vi "Error Test Label Name.vi"(6 "error text in":string, 7 "reset (F)":bool, 8 "error in":errorcluster, 10 "label name":string) -> (0 "error out":errorcluster)   [LabVIEW 2020]
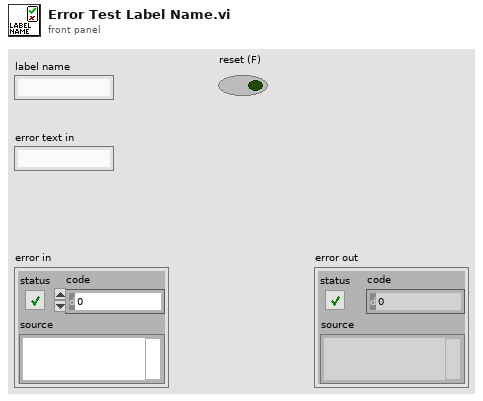
[diagram p1: front panel]
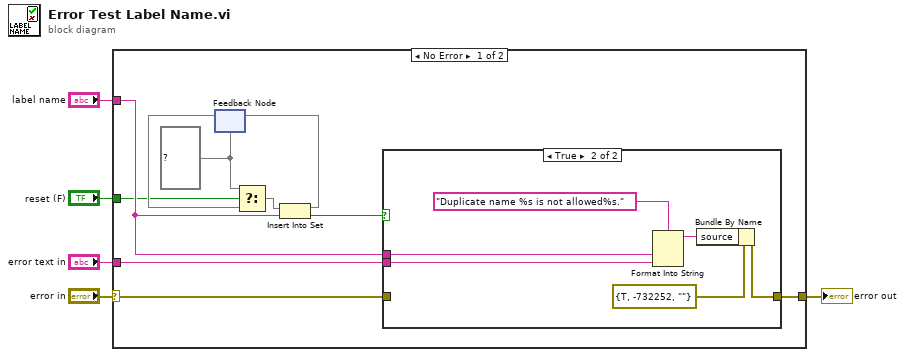
[diagram p0: block diagram]
diagram:
  n1 = case shown="No Error" "error in" {
    selector: "error in" -> [w14 w23]
    tunnel: [w13 w23] -> w4
    tunnel: "label name" -> [w15 _]
    tunnel: "reset (F)" -> [w7 _]
    tunnel: "error text in" -> [w6 _]
    frame No Error {
      w8 = set{string} {} ("set in")
      n2 = feedback #1(w8) -> (w10:set{string})
      n3 = Select(t=w8, s=w7, f=w10) -> (s? t:f=w9:set{string})
      n4 = Insert Into Set(10:w15, 11:w9) -> (2:w11:bool, 3:w12:set{string})
      n5 = feedback-in #1(w12) -> ()
      n6 = case shown="True" w11 {
        tunnel: w14 -> [w16 _]
        tunnel: [w16 w19] -> w13
        tunnel: w15 -> [_ w21]
        tunnel: w6 -> [_ w17]
        frame False {
        }
        frame True {
          n7 = Format Into String(format string="Duplicate name %s is not allowed%s." ("source"), w21, w17) -> (resulting string=w22:string)  [unwired: 2 in, 1 out]
          n8 = Bundle By Name(cluster=errorcluster {"status"=TRUE, "code"=-732252, "source"=""} ("error constant"), "source"=w22) -> (w19:errorcluster)
        }
      }
    }
    frame Error {
    }
  }
  "error out" <- w4
